vi "FindAngleDifference.vi"(10 "AngleEncoder":dbl, 11 "AngleSetpoint":dbl) -> (3 "Distance/DirectionOfTurn":dbl)   [LabVIEW 2017]
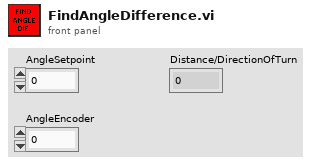
[diagram p1: front panel]
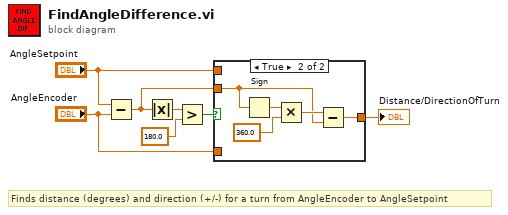
[diagram p0: block diagram]
diagram:
  # "Finds distance (degrees) and direction (+/-) for a turn from AngleEncoder to AngleSetpoint"
  n1 = Subtract(x="AngleSetpoint", y="AngleEncoder") -> (x-y=w4:dbl)
  n2 = Absolute Value(x=w4) -> (abs(x)=w5:dbl)
  n3 = Greater?(x=w5, y=180.0) -> (0:w6:bool)
  n4 = case shown="True" w6 {
    tunnel: "AngleSetpoint" -> [_ _]
    tunnel: "AngleEncoder" -> [_ _]
    tunnel: [w8 w9] -> w1
    tunnel: w4 -> [w8 w10]
    frame False {
    }
    frame True {
      n5 = Sign(1:w10) -> (0:w13:dbl)
      n6 = Multiply(x=w13, y=360.0) -> (x*y=w11:dbl)
      n7 = Subtract(x=w11, y=w10) -> (x-y=w9:dbl)
    }
  }
  "Distance/DirectionOfTurn" <- w1
